vi "Shutdown.vi"(8 "error in (no error)":errorcluster, 11 "VISA resource name":refnum<visa-resource-name>) -> (0 "error out":errorcluster, 3 "VISA resource name out":refnum<visa-resource-name>)   [LabVIEW 2020, in "Agilent ENA Series.lvlib"]
doc: "Turns off the E5070B/E5071B/E5071C."
uses:
  <instrlib>/Agilent ENA Series/Agilent ENA Series.lvlib
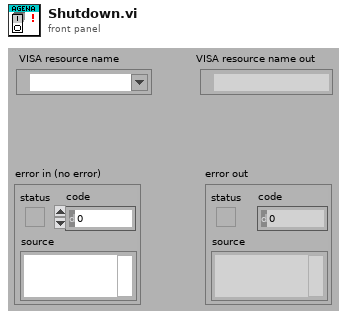
[diagram p1: front panel]
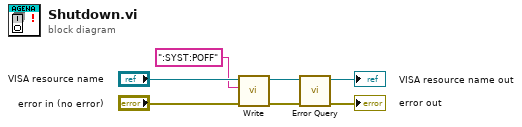
[diagram p0: block diagram]
diagram:
  n1 = call <instrlib>:"Write.vi"("error in (no error)"="error in (no error)", "String ()"=":SYST:POFF" ("format string"), "VISA resource name"="VISA resource name") -> ("error out"=w3:errorcluster, "VISA resource name out"=w4:refnum<visa-resource-name>)  [unwired: 6 in, 1 out]
  n2 = call <instrlib>:"Error Query.vi"("error in (no error)"=w3, "VISA resource name"=w4) -> ("error out"=→"error out":errorcluster, "VISA resource name out"=→"VISA resource name out":refnum<visa-resource-name>)  [unwired: 6 in, 2 out]
